vi "Isolate Table Elements.vi"(8 "Error In":errorcluster, 9 "Corner Mask":T1(plugin-control), 10 "Blue Channel In":T1(plugin-control), 11 "Red Channel In":T1(plugin-control)) -> (0 "Error Out":errorcluster, 1 "Game Ball":T1(plugin-control), 2 "Blue Team":T1(plugin-control), 3 "Red Team":T1(plugin-control))   [LabVIEW 2018]
uses:
  <vilib>/vision/NI_Vision_Development_Module.lvlib
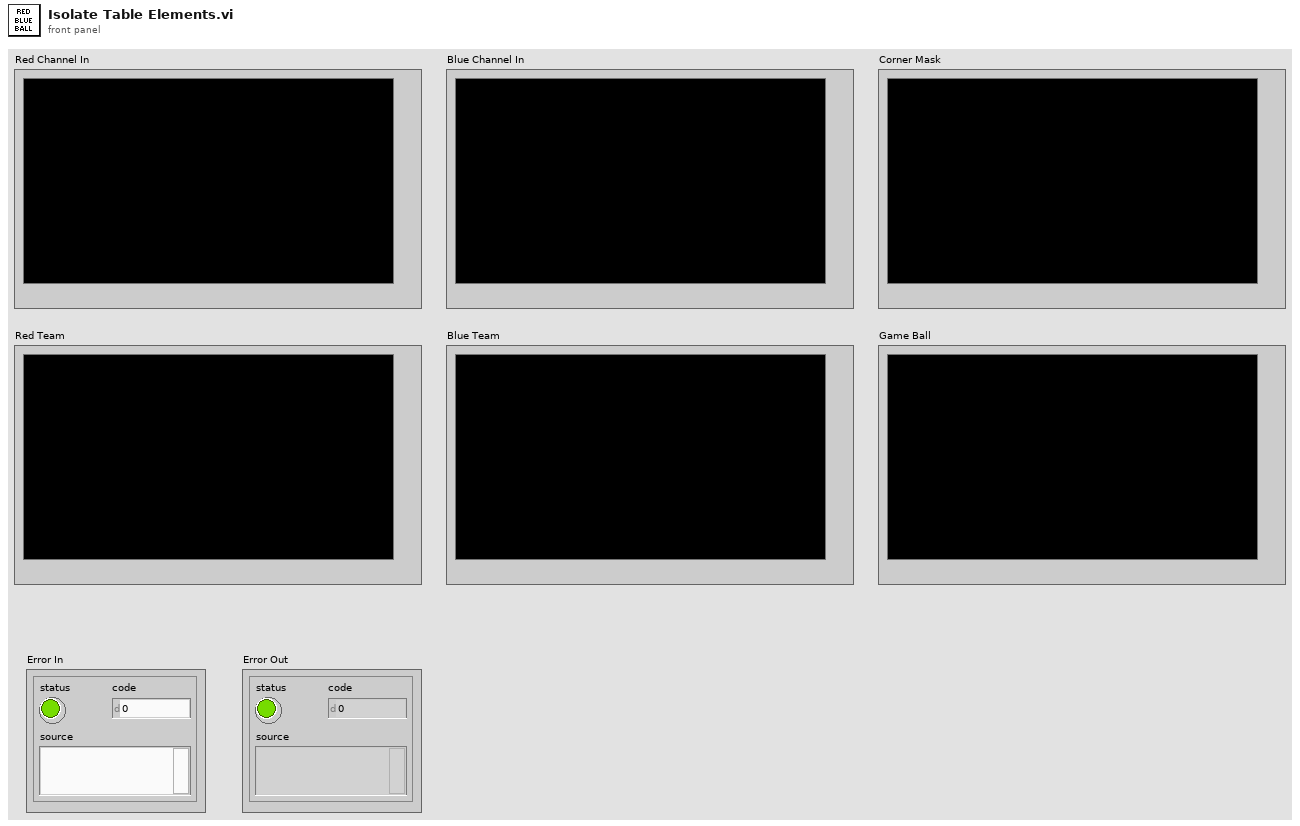
[diagram p1: front panel]
types:
  T1 = typedef "IMAQ Image.ctl" = refnum<image>
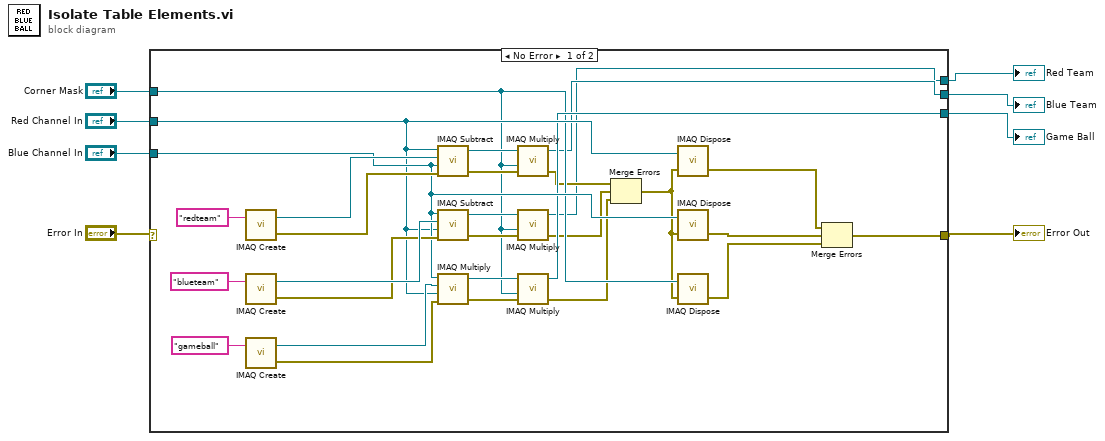
[diagram p0: block diagram]
diagram:
  n1 = case shown="No Error" "Error In" {
    selector: "Error In" -> [_ w38]
    tunnel: "Blue Channel In" -> [w22 _]
    tunnel: "Red Channel In" -> [w21 _]
    tunnel: "Corner Mask" -> [w15 _]
    tunnel: [w9 _] -> w4
    tunnel: [w10 _] -> w3
    tunnel: [w20 _] -> w2
    tunnel: [w16 w38] -> w1
    frame No Error {
      n2 = call "IMAQ Create"("Image Name"="redteam") -> ("New Image"=w34:T1, "error out"=w33:errorcluster)  [unwired: 4 in]
      n3 = call "IMAQ Create"("Image Name"="blueteam") -> ("New Image"=w32:T1, "error out"=w31:errorcluster)  [unwired: 4 in]
      n4 = call "IMAQ Create"("Image Name"="gameball") -> ("New Image"=w30:T1, "error out"=w29:errorcluster)  [unwired: 4 in]
      n5 = call "IMAQ Subtract"("Image Src A"=w21, "Image Dst"=w34, "Image Src B"=w22, "error in (no error)"=w33) -> ("Image Dst Out"=w25:T1, "error out"=w28:errorcluster)  [unwired: 3 in]
      n6 = call "IMAQ Subtract"("Image Src A"=w22, "Image Dst"=w32, "Image Src B"=w21, "error in (no error)"=w31) -> ("Image Dst Out"=w24:T1, "error out"=w27:errorcluster)  [unwired: 3 in]
      n7 = call "IMAQ Multiply"("Image Src A"=w22, "Image Dst"=w30, "Image Src B"=w21, "error in (no error)"=w29) -> ("Image Dst Out"=w23:T1, "error out"=w26:errorcluster)  [unwired: 3 in]
      n8 = call "IMAQ Multiply"("Image Src A"=w25, "Image Src B"=w15, "error in (no error)"=w28) -> ("Image Dst Out"=w10:T1, "error out"=w13:errorcluster)  [unwired: 4 in]
      n9 = call "IMAQ Multiply"("Image Src A"=w24, "Image Src B"=w15, "error in (no error)"=w27) -> ("Image Dst Out"=w9:T1, "error out"=w12:errorcluster)  [unwired: 4 in]
      n10 = call "IMAQ Multiply"("Image Src A"=w23, "Image Src B"=w15, "error in (no error)"=w26) -> ("Image Dst Out"=w20:T1, "error out"=w11:errorcluster)  [unwired: 4 in]
      n11 = Merge Errors(w13, w12, w11) -> (w14:errorcluster)
      n12 = call "IMAQ Dispose"("Image"=w21, "error in (no error)"=w14) -> ("error out"=w19:errorcluster)  [unwired: 4 in]
      n13 = call "IMAQ Dispose"("Image"=w22, "error in (no error)"=w14) -> ("error out"=w18:errorcluster)  [unwired: 4 in]
      n14 = call "IMAQ Dispose"("Image"=w15, "error in (no error)"=w14) -> ("error out"=w17:errorcluster)  [unwired: 4 in]
      n15 = Merge Errors(w19, w18, w17) -> (w16:errorcluster)
    }
    frame Error {
    }
  }
  "Error Out" <- w1
  "Red Team" <- w4
  "Blue Team" <- w3
  "Game Ball" <- w2
